vi "时间随机数查找表生成.vi"   [LabVIEW 2013]
uses:
  <vilib>/Utility/file.llb/Write To Spreadsheet File (I64).vi
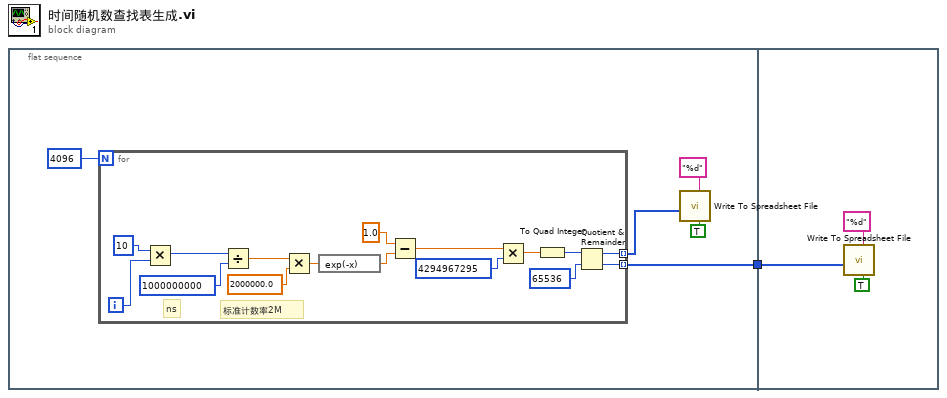
[diagram p0: block diagram]
diagram:
  n1 = flat-sequence {
    tunnel: [w2] -> w1
    tunnel: w1 -> [w23]
    frame #0 {
      n2 = for {
        N: 4096 -> [_]
        tunnel: [w10] -> w3 mode=indexing
        tunnel: [w9] -> w2 mode=indexing
        i -> [w22]
        # "标准计数率2M"
        # "ns"
        n3 = Multiply(x=i64 10, y=w22) -> (x*y=w20:i64)
        n4 = Divide(x=w20, y=i64 1000000000) -> (x/y=w16:dbl)
        n5 = Multiply(x=w16, y=2000000.0) -> (x*y=w14:dbl)
        n6 = expression code="exp(-x)"(w14) -> (w18:dbl)
        n7 = Subtract(x=1.0, y=w18) -> (x-y=w12:dbl)
        n8 = Multiply(x=w12, y=i64 4294967295) -> (x*y=w8:dbl)
        n9 = To Quad Integer(1:w8) -> (0:w7:i64)
        n10 = Quotient & Remainder(x=w7, y=u64 65536) -> (x-y*floor(x/y)=w10:u64, floor(x/y)=w9:u64)
      }
      n11 = call-poly <vilib>:"Write To Spreadsheet File.vi"("transpose? (no:F)"=TRUE, "format (%d)"="%d" ("format (%.3f)"), "1D data"=w3) -> ()  [unwired: 5 in, 1 out]
    }
    frame #1 {
      n12 = call-poly <vilib>:"Write To Spreadsheet File.vi"("transpose? (no:F)"=TRUE, "format (%d)"="%d" ("format (%.3f)"), "1D data"=w23) -> ()  [unwired: 5 in, 1 out]
    }
  }
